vi "Write Workbook.vi"(8 "error in (no error)":errorcluster, 9 "stream":refnum<k24>, 11 "IWorkbook Reference":refnum<k24>) -> (0 "error out":errorcluster, 3 "IWorkbook Reference out":refnum<k24>)   [LabVIEW 2013]
uses:
  C:/PhaeronGit/LVNPOI/Resources/NPOI 2.1.1 dotnet2/NPOI.dll
  Resources/NPOI 2.1.1 dotnet2/NPOI.dll
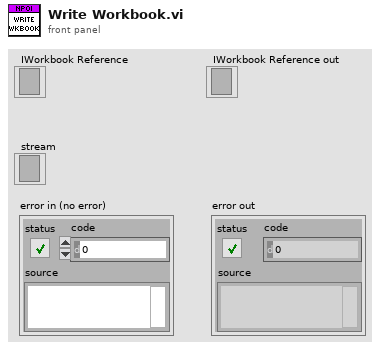
[diagram p1: front panel]
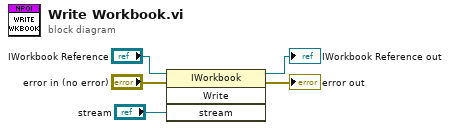
[diagram p0: block diagram]
diagram:
  n1 = invoke class="IWorkbook" method="Write"(reference="IWorkbook Reference", error in="error in (no error)", "stream"="stream") -> (reference out=→"IWorkbook Reference out":refnum<k24>, error out=→"error out":errorcluster)  [unwired: 1 in, 2 out]
